vi "getWriteTagBusRef.vi"(8 "error in":errorcluster) -> (0 "error out":errorcluster, 1 "valid references":bool, 2 "write tx data table":refnum<queue>, 3 "write data dictionary":refnum<queue>, 5 "actual write data table":refnum<queue>)   [LabVIEW 2013]
uses:
  <vilib>/NI/Tag Bus/dictionary/data dictionary.lvclass
  <vilib>/NI/Tag Bus/table/data table.ctl
  <vilib>/NI/Tag Bus/table/data table.lvlib
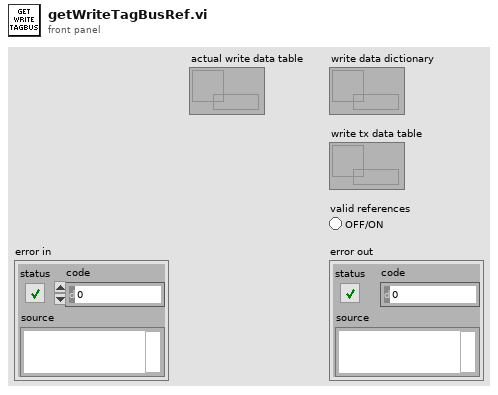
[diagram p1: front panel]
types:
  T1 = typedef "tag bus.lvlib/data table.lvlib/data table.ctl" = cluster{"Double":dbl[], "Single":sgl[], "I64":i64[], "I32":i32[], "I16":i16[], "I8":i8[], "U64":u64[], "U32":u32[], "U16":u16[], "U8":u8[], "Boolean":bool[], "String":string[], "Array of Double":cluster{"DBL Array":dbl[]}[], "Array of Single":cluster{"SGL Array":sgl[]}[], "Array of I64":cluster{"I64 Array":i64[]}[], "Array of I32":cluster{"I32 Array":i32[]}[], "Array of I16":cluster{"I16 Array":i16[]}[], "Array of I8":cluster{"I8 Array":i8[]}[], "Array of U64":cluster{"U64 Array":u64[]}[], "Array of U32":cluster{"U32 Array":u32[]}[], "Array of U16":cluster{"U16 Array":u16[]}[], "Array of U8":cluster{"U8 Array":u8[]}[], "Array of Boolean":cluster{"Boolean Array":bool[]}[], "Array of String":cluster{"String Array":string[]}[]}
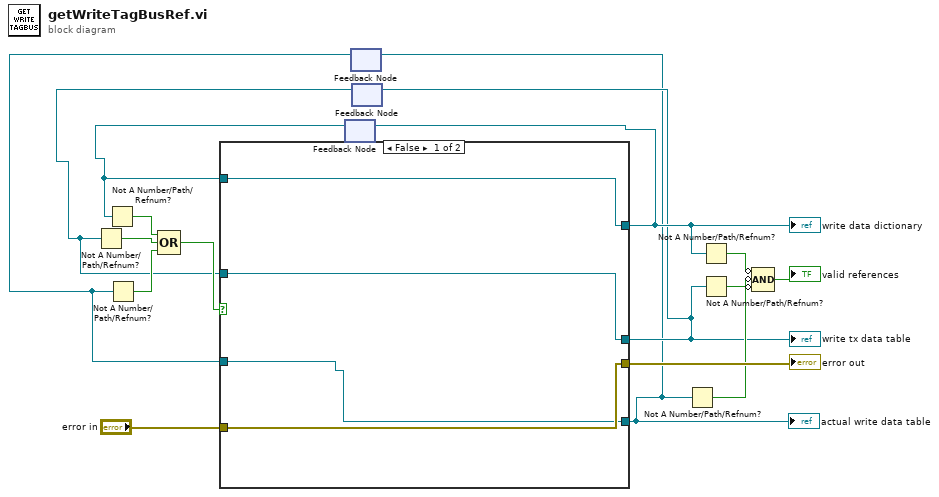
[diagram p0: block diagram]
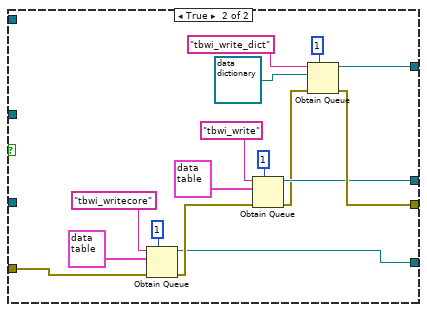
[diagram p2: hidden frame]
diagram:
  n1 = feedback #1() -> (w5:refnum<queue>)  [unwired: 1 in]
  n2 = Not A Number/Path/Refnum?(number/path/refnum=w5) -> (NaN/Path/Refnum?=w10:bool)
  n3 = feedback #2() -> (w1:refnum<queue>)  [unwired: 1 in]
  n4 = Not A Number/Path/Refnum?(number/path/refnum=w1) -> (NaN/Path/Refnum?=w8:bool)
  n5 = feedback #3() -> (w3:refnum<queue>)  [unwired: 1 in]
  n6 = Not A Number/Path/Refnum?(number/path/refnum=w3) -> (NaN/Path/Refnum?=w9:bool)
  n7 = Compound Arithmetic op=OR(w10, w9, w8) -> (w7:bool)
  n8 = case shown="False" w7 {
    tunnel: [w19 w36] -> w16
    tunnel: [w20 w35] -> w6
    tunnel: [w18 w34] -> w4
    tunnel: "error in" -> [w19 w23]
    tunnel: [w17 w21] -> w2
    tunnel: w5 -> [w20 _]
    tunnel: w3 -> [w18 _]
    tunnel: w1 -> [w17 _]
    frame False {
    }
    frame True {
      n9 = Obtain Queue(max queue size (-1, unlimited)=1, name (unnamed)="tbwi_writecore", element data type=T1 {"Double"=[], "Single"=[], "I64"=[], "I32"=[], "I16"=[], "I8"=[], "U64"=[], "U32"=[], "U16"=[], "U8"=[], "Boolean"=[], "String"=[], "Array of Double"=[], "Array of Single"=[], "Array of I64"=[], "Array of I32"=[], "Array of I16"=[], "Array of I8"=[], "Array of U64"=[], "Array of U32"=[], "Array of U16"=[], "Array of U8"=[], "Array of Boolean"=[], "Array of String"=[]} ("Data Interface out"), error in (no error)=w23) -> (queue out=w21:refnum<queue>, error out=w22:errorcluster)  [unwired: 1 in, 1 out]
      n10 = Obtain Queue(max queue size (-1, unlimited)=1, name (unnamed)="tbwi_write", element data type=T1 {"Double"=[], "Single"=[], "I64"=[], "I32"=[], "I16"=[], "I8"=[], "U64"=[], "U32"=[], "U16"=[], "U8"=[], "Boolean"=[], "String"=[], "Array of Double"=[], "Array of Single"=[], "Array of I64"=[], "Array of I32"=[], "Array of I16"=[], "Array of I8"=[], "Array of U64"=[], "Array of U32"=[], "Array of U16"=[], "Array of U8"=[], "Array of Boolean"=[], "Array of String"=[]} ("Data Interface out"), error in (no error)=w22) -> (queue out=w34:refnum<queue>, error out=w29:errorcluster)  [unwired: 1 in, 1 out]
      n11 = Obtain Queue(max queue size (-1, unlimited)=1, name (unnamed)="tbwi_write_dict", element data type=refnum<class "data dictionary.lvclass"> refnum ("input data.data dictionary"), error in (no error)=w29) -> (queue out=w35:refnum<queue>, error out=w36:errorcluster)  [unwired: 1 in, 1 out]
    }
  }
  "write data dictionary" <- w6
  "error out" <- w16
  "write tx data table" <- w4
  "actual write data table" <- w2
  n12 = feedback-in #1(w6) -> ()
  n13 = feedback-in #2(w2) -> ()
  n14 = feedback-in #3(w4) -> ()
  n15 = Not A Number/Path/Refnum?(number/path/refnum=w2) -> (NaN/Path/Refnum?=w11:bool)
  n16 = Not A Number/Path/Refnum?(number/path/refnum=w6) -> (NaN/Path/Refnum?=w14:bool)
  n17 = Not A Number/Path/Refnum?(number/path/refnum=w4) -> (NaN/Path/Refnum?=w15:bool)
  n18 = Compound Arithmetic op=AND(invert w14, invert w15, invert w11) -> (→"valid references":bool)
